vi "Configure 2Wire Resistance.vi"(0 "VISA resource name":refnum<visa-resource-name>, 1 "Set Aperture or NPLC? (T: Aperture)":bool, 5 "Auto Range? (T: Auto)":bool, 7 "Manual Range":dbl=1000.0, 9 "Aperture Seconds":dbl=0.01616, 11 "error in (no error)":errorcluster) -> (4 "VISA resource name out":refnum<visa-resource-name>, 15 "error out":errorcluster)   [LabVIEW 2018, in "Keithley DMM7512.lvlib"]
doc: "This VI configures the 2 wire Resistance."
uses:
  <instrlib>/Keithley DMM7512/Keithley DMM7512.lvlib
panel:
  in  "NPLC":dbl=1.0 min=0.0005 max=15.0 step=1.0
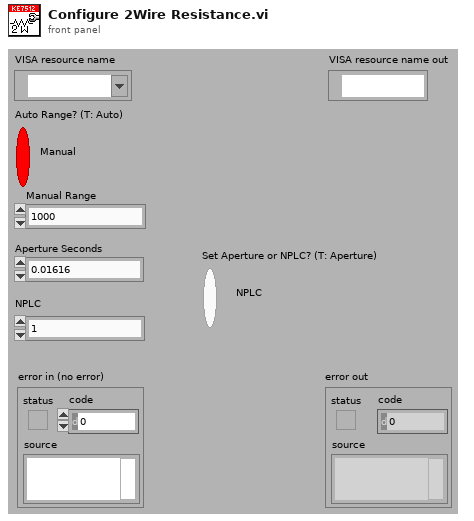
[diagram p1: front panel]
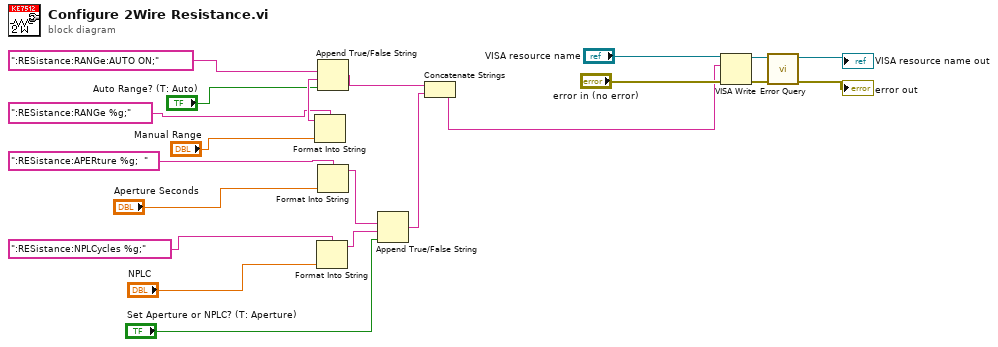
[diagram p0: block diagram]
diagram:
  n1 = Format Into String(format string=":RESistance:RANGe %g;", "Manual Range") -> (resulting string=w14:string)  [unwired: 2 in, 1 out]
  n2 = Format Into String(format string=":RESistance:NPLCycles %g;", "NPLC") -> (resulting string=w4:string)  [unwired: 2 in, 1 out]
  n3 = Append True/False String(1:"Auto Range? (T: Auto)", 2:w14, 3:":RESistance:RANGe:AUTO ON;") -> (0:w13:string)  [unwired: 1 in]
  n4 = Format Into String(format string=":RESistance:APERture %g;  ", "Aperture Seconds") -> (resulting string=w6:string)  [unwired: 2 in, 1 out]
  n5 = Append True/False String(1:"Set Aperture or NPLC? (T: Aperture)", 2:w4, 3:w6) -> (0:w7:string)  [unwired: 1 in]
  n6 = Concatenate Strings(w13, w7) -> (w12:string)
  n7 = VISA Write(VISA resource name="VISA resource name", write buffer=w12, error in (no error)="error in (no error)") -> (VISA resource name out=w21:refnum<visa-resource-name>, error out=w20:errorcluster)  [unwired: 1 out]
  n8 = call <instrlib>:"Error Query.vi"("error in (no error)"=w20, "VISA resource name"=w21) -> ("error out"=→"error out":errorcluster, "VISA resource name out"=→"VISA resource name out":refnum<visa-resource-name>)  [unwired: 6 in, 2 out]
